vi "FRIC_navX_Internal_SPI_ProcessingLoop.vi"(7 "Device Number":T2, 11 "Rate (4Hz-200Hz)":u8=50 min=4 max=200) -> ()   [LabVIEW 2016, in "navX Library.lvlib"]
doc: "This navX VI handles the reading/writing for the navX. All of the good stuff is in here.\nTHIS VI SHOULD NOT BE CALLED BY THE USER!"
uses:
  navX Library.lvlib
  <vilib>/Rock Robotics/SystemInterfaces/spilib/spi_bus.ctl
  _TypeDefs/FRIC_navX_DeviceNumbersTypeDef.ctl
  _TypeDefs/FRIC_navX_I2C Process Loop TypeDef.ctl
  _TypeDefs/FRIC_navX_ProcessingLoopStatesTypeDef_I2C.ctl
  _TypeDefs/Z900_navX_DeviceTypeDef.ctl
  _TypeDefs/Z900_navX_ProtocolTypeDef.ctl
  _TypeDefs/Z900_navX_NotifyPacketTypeDef.ctl
  _TypeDefs/Z900_navX_ActionTypeDef.ctl
  _TypeDefs/Z900_navX_SerialStreamTypeDef.ctl
  <vilib>/Rock Robotics/SystemInterfaces/i2clib/i2c_bus.ctl
  _TypeDefs/Z900_navX_IntegrationControlRegisters.ctl
  <vilib>/Rock Robotics/WPI/SPI/WPI_SPIDevRef.ctl
  <vilib>/Rock Robotics/WPI/SerialPort/WPI_SerialPort.ctl
  <vilib>/Rock Robotics/WPI/SerialPort/WPI_SerialPortRef.ctl
  <vilib>/Platform/TimedLoop/XDataNode/timing_clust.ctl
  <vilib>/Platform/TimedLoop/XDataNode/nitl_modes.ctl
  <vilib>/Platform/TimedLoop/XDataNode/wakeup.ctl
  _TypeDefs/Flags/Z900_navX_Flags_CapabilityTypeDef.ctl
  _TypeDefs/Z900_navX_DeviceRegisters.ctl
  _Util/Z900_navX_Util_LittleEndian_to_BigEndian.vi
  <vilib>/Rock Robotics/SystemInterfaces/Utilities/FPGA_UtilitiesRead LocalTime.vi
  <vilib>/Platform/TimedLoop/XDataNode/XDataNode.xnode
  <vilib>/Platform/TimedLoop/XDataNode/XDNodeRunTimeDep.lvlib
panel:
  in  "Tab Control":enum32{"Page 1", "Page 2"}(tab)
  in  "Halt":bool
  out "Connected":bool
  in  "SPI Bus":T1=enum."SPI MXP"
  in  "Clock Rate (Hz)":dbl=2000000.0 format="%_6f"
  out "error":errorcluster
  out "Loop dt":i64
  out "Loop TIme":i64
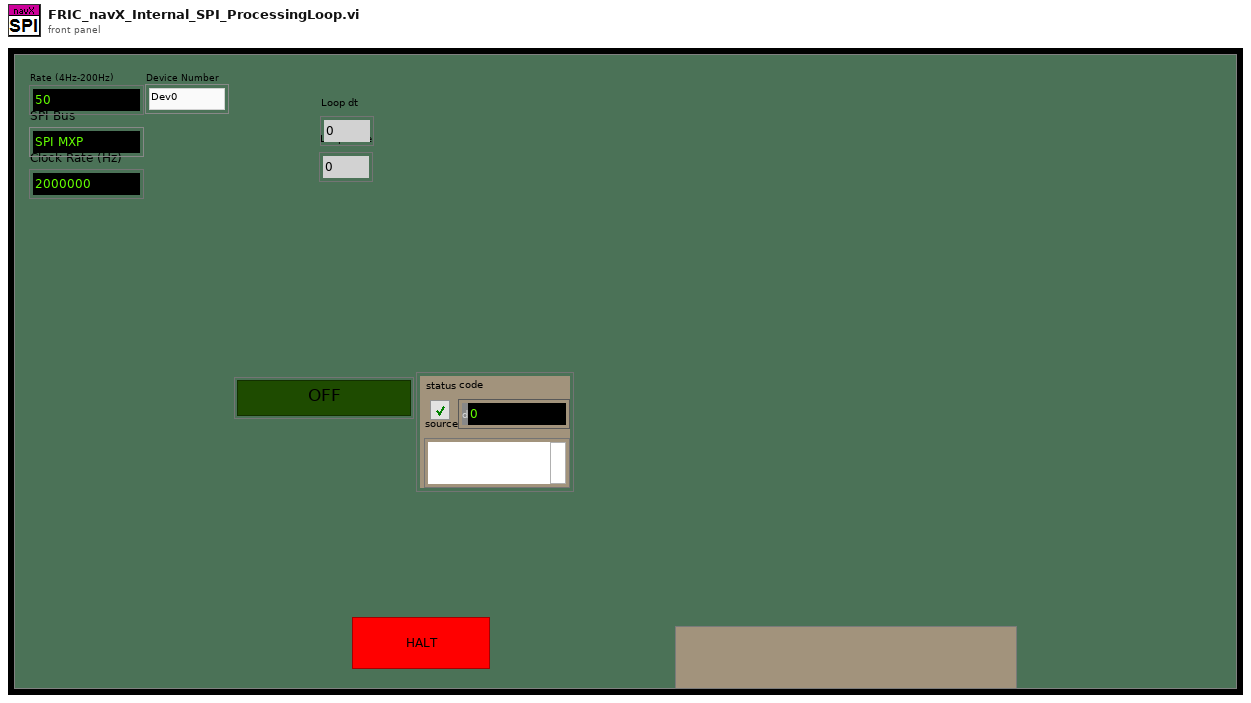
[diagram p1: front panel]
types:
  T1 = typedef "spi_bus.ctl" = enum16{"SPI On-Board, CS0", "SPI On-Board, CS1", "SPI On-Board, CS2", "SPI On-Board, CS3", "SPI MXP", "Invalid"}
  T2 = typedef "navX Library.lvlib/FRIC_navX_DeviceNumbersTypeDef.ctl" = enum16{"Dev0", "Dev1", "Dev2", "Dev3"}
  T3 = typedef "navX Library.lvlib/FRIC_navX_I2C Process Loop TypeDef.ctl" = cluster{"State Array":T4[], "error":errorcluster, "FPGA Cluster":cluster{"Last Valid FPGA Time":dbl, "Error Count":i32, "Initialized":bool}, "Device Info":T5, "I2CDevRef":cluster{"DevStatus":errorcluster, "Device Address":u8, "Handle":i32, "I2C Bus":T7}, "Registry":u8[], "Command Array":T8[], "Connected?":bool, "navX Device Memory Size":i32, "notification":T9, "Memory Size Set":bool, "SPIDevRef":T12, "navX Serial Open":cluster{"Stream Type":T11, "Serial Port":T13}, "SerialPortRef":T14, "Serial Read Buffer":string, "Serial Write Buffer":string[], "Device Number":T2, "navX SPI Open":cluster{"SPI Bus":T1, "Clock Rate (Hz)":dbl}, "Loop dt":i64, "current time":timestamp, "Loop Time":i64}
  T4 = typedef "navX Library.lvlib/FRIC_navX_ProcessingLoopStatesTypeDef_I2C.ctl" = enum16{"Process", "INI", "Check Packets Valid", "Close", "Clear VISA", "Generate Command", "Last Packet Valid", "Open", "Read", "Reset Serial", "Set Termination Char", "Update AE", "Wait", "Write", "Exit"}
  T5 = typedef "navX Library.lvlib/Z900_navX_DeviceTypeDef.ctl" = cluster{"Interface":cluster{"Protocol":T6, "Update Rate (4Hz-200Hz)":u8, "navX Open TypeDef":variant}, "Notify Packet":refnum<notifier>, "Loop VI Refnum":refnum<vi>, "Ready to Close Occurrence Refnum":refnum<k4>, "Name":string}
  T6 = typedef "navX Library.lvlib/Z900_navX_ProtocolTypeDef.ctl" = enum16{"SERIAL", "I2C", "SPI"}
  T7 = typedef "i2c_bus.ctl" = enum16{"I2C On-Board", "I2C MXP", "Invalid"}
  T8 = typedef "navX Library.lvlib/Z900_navX_IntegrationControlRegisters.ctl" = u8
  T9 = typedef "navX Library.lvlib/Z900_navX_NotifyPacketTypeDef.ctl" = cluster{"navX Action":T10, "Data":variant, "Stream Type":T11, "Device Number":T2}
  T10 = typedef "navX Library.lvlib/Z900_navX_ActionTypeDef.ctl" = enum16{"None", "Halt", "Normal Read", "Update Serial Protocol", "Update Rate Htz", "Zero-Yaw", "Zero-Displacement", "Zero-Velocity"}
  T11 = typedef "navX Library.lvlib/Z900_navX_SerialStreamTypeDef.ctl" = enum16{"YRPH", "Quaterinons", "Gyro/Raw", "AHRS", "AHRSAndPositioning", "AHRSAndPOSTime"}
  T12 = typedef "WPI_SPIDevRef.ctl" = cluster{"DevStatus":errorcluster, "Handle":i32, "SPI Bus":T1}
  T13 = typedef "WPI_SerialPort.ctl" = enum16{"Onboard RS-232", "MXP TTL", "USB 1", "USB 2"}
  T14 = typedef "WPI_SerialPortRef.ctl" = cluster{"DevStatus":errorcluster, "Serial Port Name":refnum<visa-resource-name>}
  T15 = typedef "XDNodeRunTimeDep.lvlib/timing_clust.ctl" = cluster{"Expected End [f-1]":u64, "Actual End [f-1]":u64, "Finished Late? [f-1]":bool, "Expected End [i-1]":u64, "Actual End [i-1]":u64, "Finished Late? [i-1]":bool, "Expected Start [i]":u64, "Actual Start [i]":u64, "Expected Start [f]":u64, "Actual Start [f]":u64, "Source Name":string, "Structure Name":string, "Period":i64, "Deadline":i64, "Offset":i64, "Start":i64, "Priority":i32, "Timeout":i32, "Mode":T16, "Wakeup Reason":T17, "Error":errorcluster, "Source Type":string, "Secondary Source Type":string, "Global End Time":u64, "Global Start Time":u64, "Frame Duration":u64, "Iteration Duration":u64, "Assigned CPU":i32, "I/O Scan Engine Mode":u32}
  T16 = typedef "XDNodeRunTimeDep.lvlib/nitl_modes.ctl" = enum32{"No Change", "Process missed periods, maintain original phase", "Discard missed periods, maintain original phase", "Process missed periods, ignore original phase", "Discard missed periods, ignore original phase"}
  T17 = typedef "XDNodeRunTimeDep.lvlib/wakeup.ctl" = enum32{"Normal", "Aborted", "Asynchronous wakeup", "Timing source error", "Timed loop error", "Timeout"}
  T18 = typedef "navX Library.lvlib/Z900_navX_DeviceRegisters.ctl" = u8
  T19 = typedef "navX Library.lvlib/Z900_navX_Flags_CapabilityTypeDef.ctl" = u16
  T20 = cluster{"Last Valid FPGA Time":dbl, "Error Count":i32, "Initialized":bool}
  T21 = typedef "Z900_navX_NotifyPacketTypeDef.ctl" = cluster{"navX Action":T22, "Data":variant, "Stream Type":T23, "Device Number":T24}
  T22 = typedef "Z900_navX_ActionTypeDef.ctl" = enum16{"None", "Halt", "Normal Read", "Update Serial Protocol", "Update Rate Htz", "Zero-Yaw", "Zero-Displacement", "Zero-Velocity"}
  T23 = typedef "Z900_navX_SerialStreamTypeDef.ctl" = enum16{"YRPH", "Quaterinons", "Gyro/Raw", "AHRS", "AHRSAndPositioning", "AHRSAndPOSTime"}
  T24 = typedef "FRIC_navX_DeviceNumbersTypeDef.ctl" = enum16{"Dev0", "Dev1", "Dev2", "Dev3"}
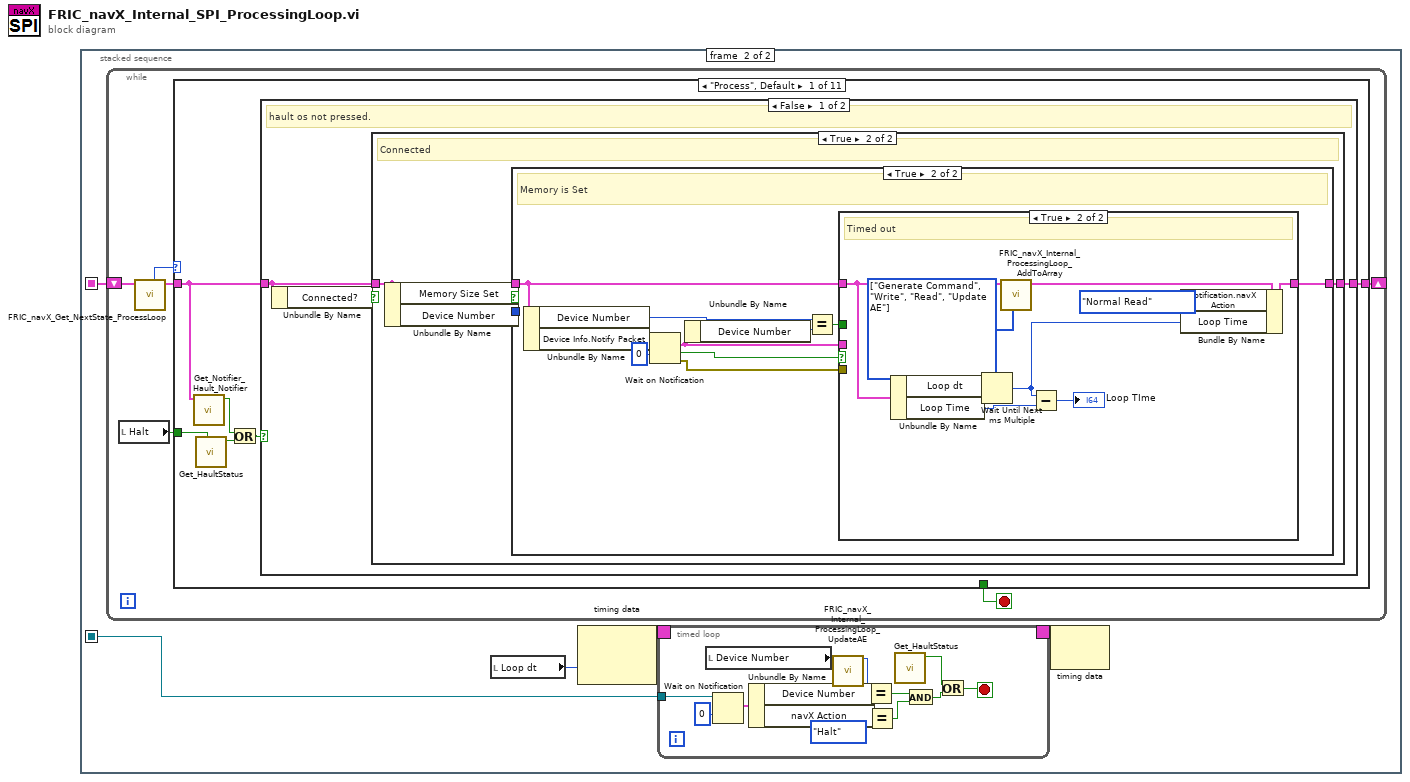
[diagram p0: block diagram]
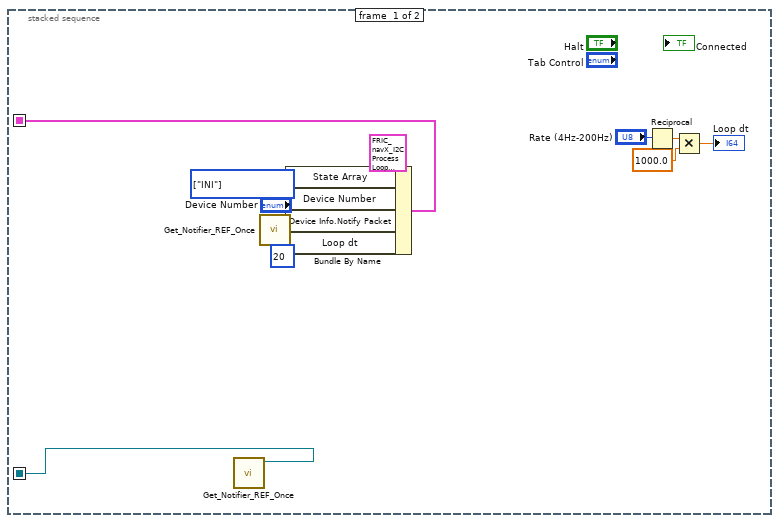
[diagram p2: hidden frame]
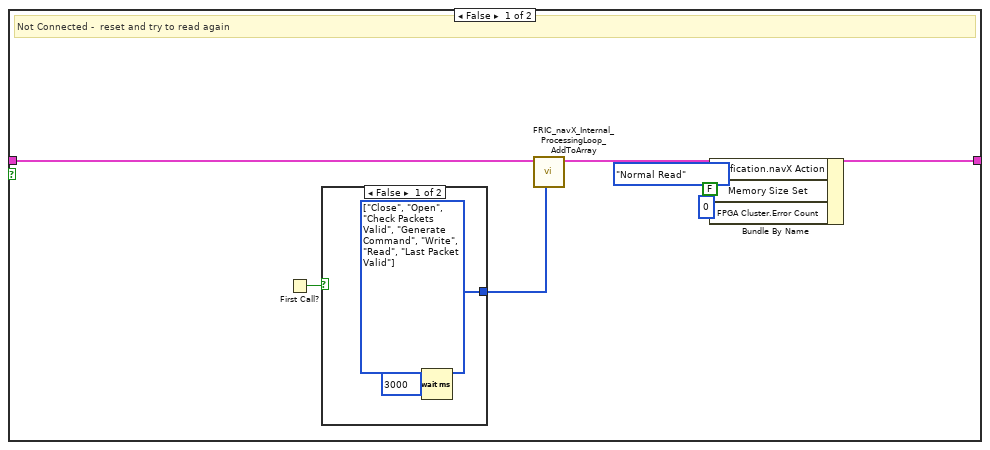
[diagram p3: hidden frame]
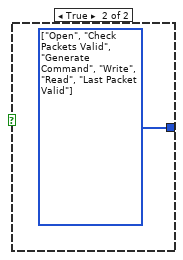
[diagram p4: hidden frame]
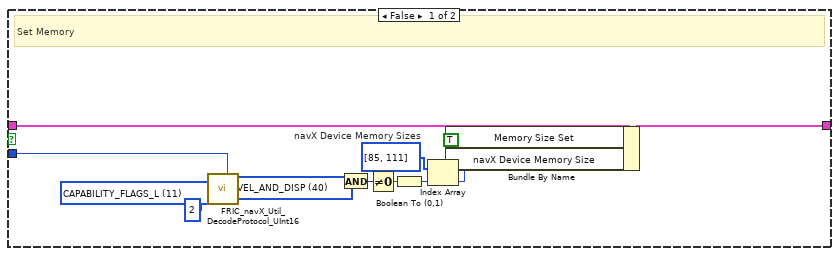
[diagram p5: hidden frame]
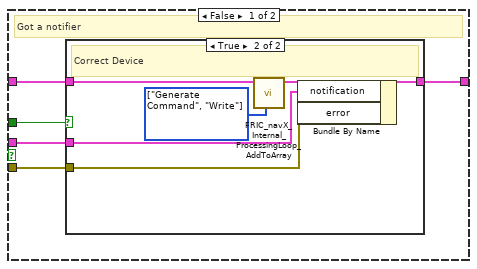
[diagram p6: hidden frame]
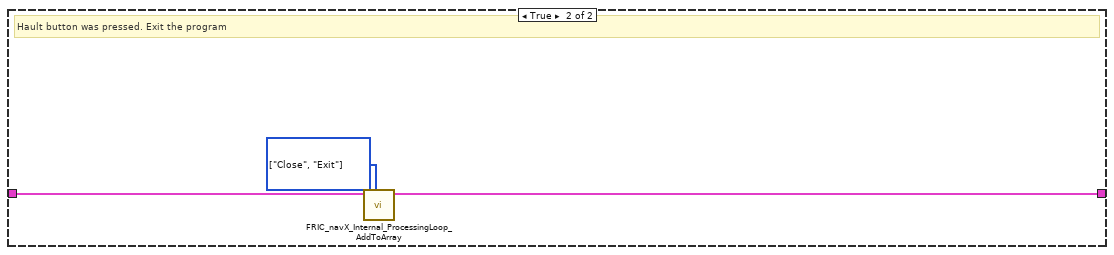
[diagram p8: hidden frame]
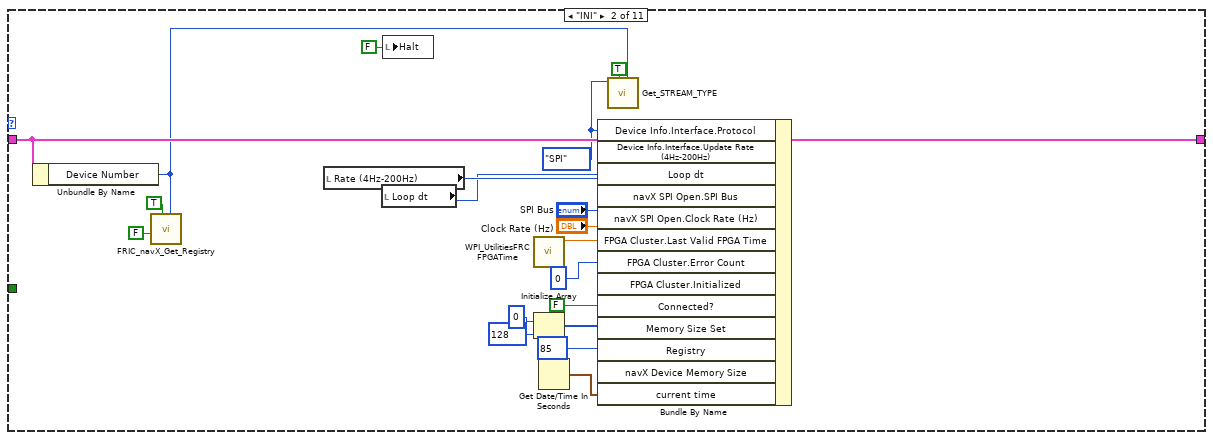
[diagram p9: hidden frame]
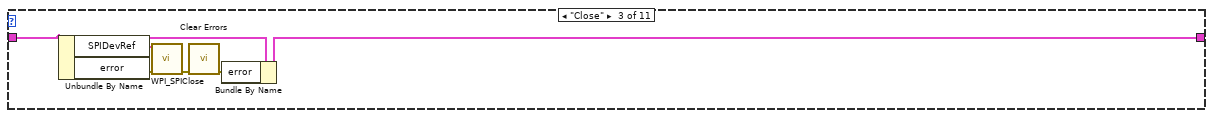
[diagram p10: hidden frame]
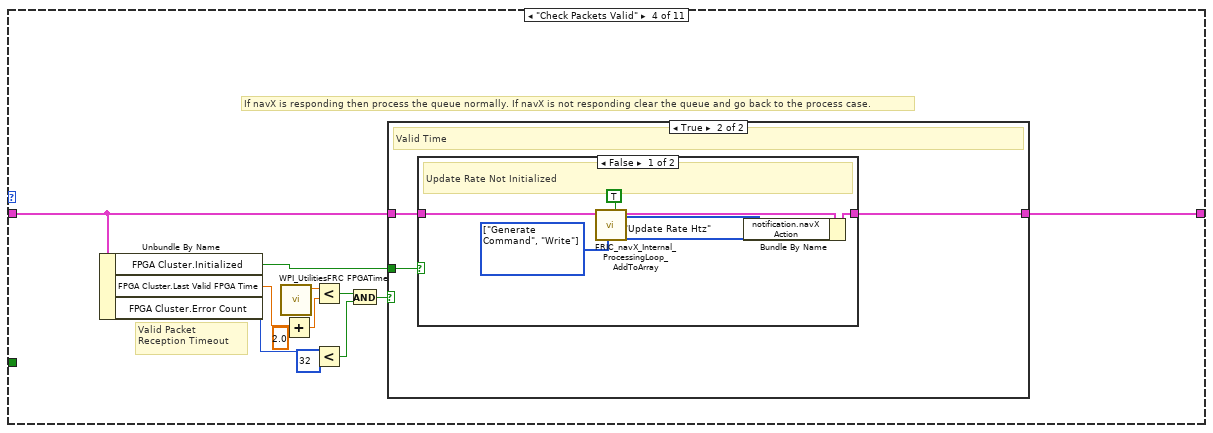
[diagram p11: hidden frame]
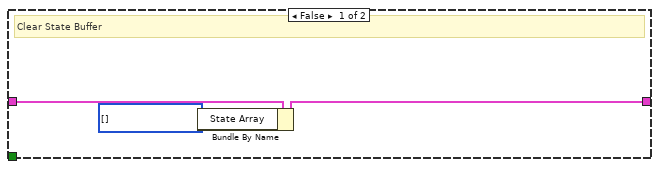
[diagram p12: hidden frame]
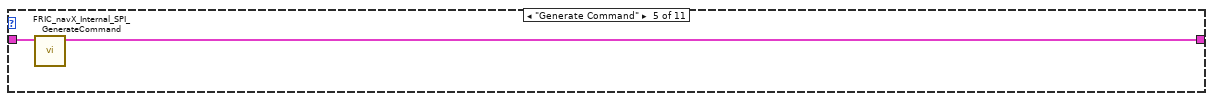
[diagram p14: hidden frame]
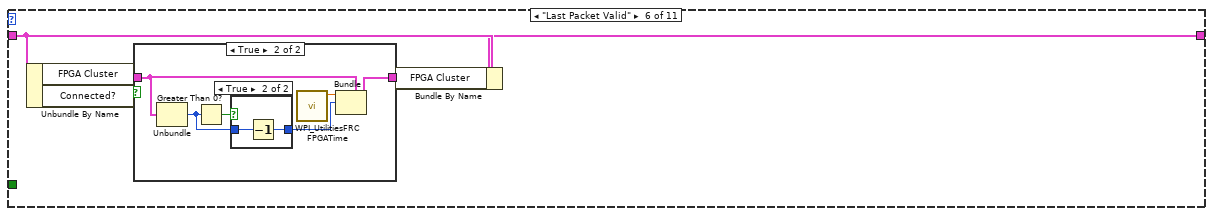
[diagram p15: hidden frame]
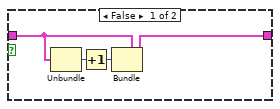
[diagram p16: hidden frame]
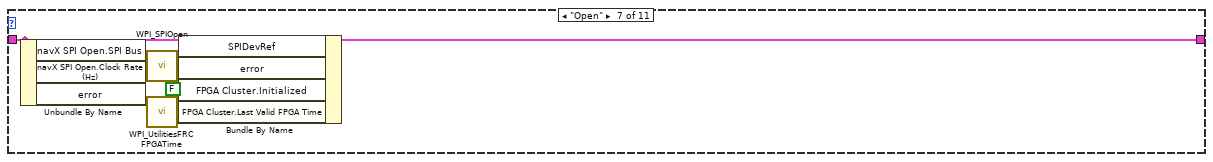
[diagram p18: hidden frame]
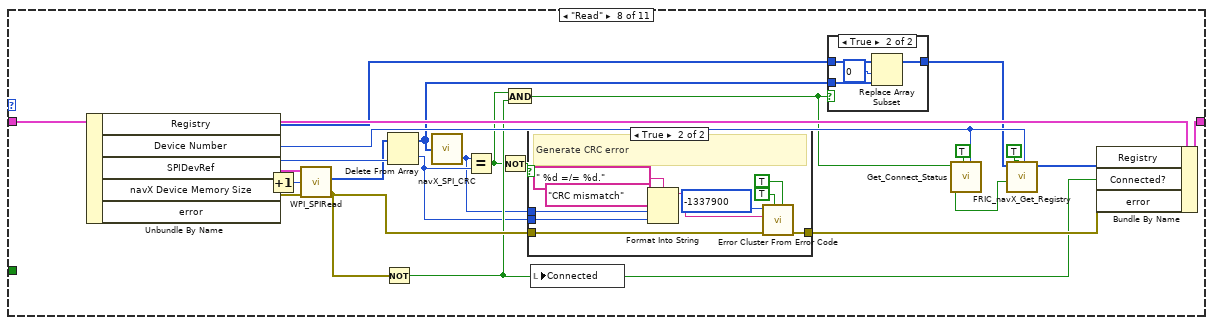
[diagram p19: hidden frame]
diagram:
  n1 = stacked-sequence {
    seq-local: [w11 _] -> [_ w16]
    seq-local: [w5 _] -> [_ w15]
    frame #0 {
      w9 = T4[] [enum."INI"] items=["Process", "INI", "Check Packets Valid", "Close", "Clear VISA", "Generate Command", "Last Packet Valid", "Open", "Read", "Reset Serial", "Set Termination Char", "Update AE", "Wait", "Write", "Exit"] ("State Array")
      n2 = call "Get_Notifier_REF_Once.vi"() -> ("notifier ref out"=w5:refnum<notifier>)  [unwired: 10 in, 1 out]
      n3 = call "Get_Notifier_REF_Once.vi"() -> ("notifier ref out"=w7:refnum<notifier>)  [unwired: 10 in, 1 out]
      n4 = Bundle By Name(cluster=T3 {"State Array"=[enum."INI", enum."Open"], "error"={"status"=FALSE, "code"=0, "source"=""}, "FPGA Cluster"={"Last Valid FPGA Time"=0.0, "Error Count"=0, "Initialized"=FALSE}, "Device Info"={"Interface"={"Protocol"=enum."SERIAL", "Update Rate (4Hz-200Hz)"=4, "navX Open TypeDef"=variant}, "Notify Packet"=refnum, "Loop VI Refnum"=refnum, "Ready to Close Occurrence Refnum"=refnum, "Name"=""}, "I2CDevRef"={"DevStatus"={"status"=FALSE, "code"=0, "source"=""}, "Device Address"=0, "Handle"=0, "I2C Bus"=enum."Invalid"}, "Registry"=[], "Command Array"=[214, 32], "Connected?"=FALSE, "navX Device Memory Size"=85, "notification"={"navX Action"=enum."None", "Data"=variant, "Stream Type"=enum."YRPH", "Device Number"=enum."Dev0"}, "Memory Size Set"=FALSE, "SPIDevRef"={"DevStatus"={"status"=FALSE, "code"=0, "source"=""}, "Handle"=0, "SPI Bus"=enum."SPI On-Board, CS0"}, "navX Serial Open"={"Stream Type"=enum."YRPH", "Serial Port"=enum."Onboard RS-232"}, "SerialPortRef"={"DevStatus"={"status"=FALSE, "code"=0, "source"=""}, "Serial Port Name"=""}, "Serial Read Buffer"="", "Serial Write Buffer"=[], "Device Number"=enum."Dev0", "navX SPI Open"={"SPI Bus"=enum."SPI MXP", "Clock Rate (Hz)"=500000.0}, "Loop dt"=0, "current time"=timestamp(0 s since 1904-01-01), "Loop Time"=0} ("I2C Process Loop TypeDef"), "State Array"=w9, "Device Number"="Device Number", "Device Info.Notify Packet"=w7, "Loop dt"=i64 20) -> (w11:T3)
      n5 = Reciprocal(x="Rate (4Hz-200Hz)") -> (1/x=w2:dbl)
      n6 = Multiply(x=w2, y=1000.0) -> (x*y=→"Loop dt":dbl)
    }
    frame #1 {
      n7 = while {
        shift-right: [w36] -> _
        shift-left: w16 -> [w39]
        stop <- w40 stop-if-true
        n8 = local read "Halt"() -> (w35:bool)
        n9 = call "FRIC_navX_Get_NextState_ProcessLoop.vi"("I2C Process Loop TypeDef (in)"=w39) -> ("I2C Process Loop TypeDef (out)"=w38:T3, "Current State"=w37:T4)  [unwired: 9 in]
        n10 = case shown="\"Process\", Default" w37 {
          tunnel: [_ _ _ _ _ _ _ _ _ w240 _] -> w40
          tunnel: w38 -> [w45 w120 w137 w141 w164 w168 w191 w213 w237 w242 w250]
          tunnel: [w46 w126 w136 w142 w163 w167 w190 w212 w230 w242 w250] -> w36
          tunnel: w35 -> [w43 _ _ _ _ _ _ _ _ _ _]
          frame "Process", Default {
            n11 = call "Get_Notifier_Hault_Notifier.vi"("Process Loop TypeDef (in)"=w45) -> ("Hault Notifier"=w41:bool)  [unwired: 10 in]
            n12 = call "Get_HaultStatus.vi"("Update"=w43) -> ("Hault"=w42:bool)  [unwired: 10 in]
            n13 = Or(x=w41, y=w42) -> (x .or. y?=w44:bool)
            n14 = case shown="False" w44 {
              tunnel: [w49 w110] -> w46
              tunnel: w45 -> [w47 w111]
              frame False {
                # "hault os not pressed."
                n15 = Unbundle By Name(w47) -> ("Connected?"=w48:bool)
                n16 = case shown="True" w48 {
                  tunnel: w47 -> [w57 w63]
                  tunnel: [w54 w64] -> w49
                  frame False {
                    # "Not Connected -  reset and try to read again"
                    n17 = First Call?() -> (First Call?: T/F=w50:bool)
                    n18 = case shown="False" w50 {
                      tunnel: [w59 w60] -> w56
                      frame False {
                        w59 = T4[] [enum."Close", enum."Open", enum."Check Packets Valid", enum."Generate Command", enum."Write", enum."Read", enum."Last Packet Valid"] items=["Process", "INI", "Check Packets Valid", "Close", "Clear VISA", "Generate Command", "Last Packet Valid", "Open", "Read", "Reset Serial", "Set Termination Char", "Update AE", "Wait", "Write", "Exit"]
                        n19 = Wait (ms)(milliseconds to wait=u32 3000) -> ()  [unwired: 1 out]
                      }
                      frame True {
                        w60 = T4[] [enum."Open", enum."Check Packets Valid", enum."Generate Command", enum."Write", enum."Read", enum."Last Packet Valid"] items=["Process", "INI", "Check Packets Valid", "Close", "Clear VISA", "Generate Command", "Last Packet Valid", "Open", "Read", "Reset Serial", "Set Termination Char", "Update AE", "Wait", "Write", "Exit"]
                      }
                    }
                    n20 = call "FRIC_navX_Internal_ProcessingLoop_AddToArray.vi"("States Array"=w56, "I2C Process Loop TypeDef (in)"=w57) -> ("I2C Process Loop TypeDef (out)"=w55:T3)  [unwired: 9 in]
                    n21 = Bundle By Name(cluster=w55, "notification.navX Action"=Z900_navX_ActionTypeDef."Normal Read", "Memory Size Set"=FALSE, "FPGA Cluster.Error Count"=0) -> (w54:T3)
                  }
                  frame True {
                    # "Connected"
                    n22 = Unbundle By Name(w63) -> ("Memory Size Set"=w62:bool, "Device Number"=w61:T2)
                    n23 = case shown="True" w62 {
                      tunnel: [w76 w85] -> w64
                      tunnel: w63 -> [w77 w83]
                      tunnel: w61 -> [w65 _]
                      frame False {
                        w75 = T18 11 items=["WHOAMI"=0, "HW_REV"=1, "FW_VER_MAJOR"=2, "FW_VER_MINOR"=3, "UPDATE_RATE_HZ"=4, "ACCEL_FSR_G"=5, "GYRO_FSR_DPS"=6, "OP_STATUS"=8, "CAL_STATUS"=9, "SELFTEST_STATUS"=10, "CAPABILITY_FLAGS_L"=11, "CAPABILITY_FLAGS_H"=12, "SENSOR_STATUS"=16, "TIMESTAMP"=18, "YAW"=22, "ROLL"=24, "PITCH"=26, "HEADING"=28, "FUSED_HEADING"=30, "ALTITUDE_I"=32, "ALTITUDE_D"=34, "LINERA_ACC_X"=36, "LINERA_ACC_Y"=38, "LINERA_ACC_Z"=40, "QUAT_W"=42, "QUAT_X"=44, "QUAT_Y"=46, "QUAT_Z"=48, "MPU_TEMP_C"=50, "GYRO_X"=52, "GYRO_Y"=54, "GYRO_Z"=56, "ACC_X"=58, "ACC_Y"=60, "ACC_Z"=62, "MAG_X"=64, "MAG_Y"=66, "MAG_Z"=68, "PRESSURE_I"=70, "PRESSURE_D"=72, "PRESSURE_TEMP"=74, "YAW_OFFSET"=76, "QUAT_OFFSET_W"=78, "QUAT_OFFSET_X"=80, "QUAT_OFFSET_Y"=82, "QUAT_OFFSET_Z"=84, "INTEGRATION_CONTROL"=86, "VELOCITY_X"=88, "VELOCITY_Y"=92, "VELOCITY_Z"=96, "DISPLACMENT_X"=100, "DISPLACMENT_Y"=104, "DISPLACEMENT_Z"=108] ("Device Register")
                        w70 = T19 40 items=["OMNIMOUNT"=4, "OMNIMOUNT_CONFIG_MASK"=38, "VEL_AND_DISP"=40, "YAW_RESET"=80] ("Capability Flag")
                        w71 = i32[] [85, 111]  # navX Device Memory Sizes
                        # "Set Memory"
                        n24 = call "FRIC_navX_Util_DecodeProtocol_UInt16.vi"("Device Number"=w65, "length"=2, "Device Register"=w75) -> ("Value"=w68:u16)  [unwired: 8 in]
                        n25 = And(x=w68, y=w70) -> (x .and. y?=w69:T19)
                        n26 = Not Equal To 0?(x=w69) -> (x != 0?=w72:bool)
                        n27 = Boolean To (0,1)(Boolean=w72) -> (0, 1=w73:i16)
                        n28 = Index Array(array=w71, index=w73) -> (element=w66:i32)
                        n29 = Bundle By Name(cluster=w77, "Memory Size Set"=TRUE, "navX Device Memory Size"=w66) -> (w76:T3)
                      }
                      frame True {
                        # "Memory is Set"
                        n30 = Unbundle By Name(w83) -> ("Device Number"=w80:T2, "Device Info.Notify Packet"=w87:refnum<notifier>)
                        n31 = Wait on Notification(notifier=w87, timeout in ms (-1)=0) -> (notification=w81:T9, timed out?=w82:bool, error out=w84:errorcluster)  [unwired: 2 in, 1 out]
                        n32 = Unbundle By Name(w81) -> ("Device Number"=w79:T2)
                        n33 = Equal?(x=w80, y=w79) -> (x = y?=w78:bool)
                        n34 = case shown="True" w82 {
                          tunnel: w83 -> [w92 w104]
                          tunnel: [w91 w106] -> w85
                          tunnel: w81 -> [w90 _]
                          tunnel: w84 -> [w89 _]
                          tunnel: w78 -> [w88 _]
                          frame False {
                            # "Got a notifier"
                            n35 = case shown="True" w88 {
                              tunnel: w92 -> [w93 w99]
                              tunnel: [w93 w98] -> w91
                              tunnel: w90 -> [_ w97]
                              tunnel: w89 -> [_ w94]
                              frame False {
                              }
                              frame True {
                                w95 = T4[] [enum."Generate Command", enum."Write"] items=["Process", "INI", "Check Packets Valid", "Close", "Clear VISA", "Generate Command", "Last Packet Valid", "Open", "Read", "Reset Serial", "Set Termination Char", "Update AE", "Wait", "Write", "Exit"] ("States Array")
                                # "Correct Device"
                                n36 = call "FRIC_navX_Internal_ProcessingLoop_AddToArray.vi"("States Array"=w95, "I2C Process Loop TypeDef (in)"=w99) -> ("I2C Process Loop TypeDef (out)"=w96:T3)  [unwired: 9 in]
                                n37 = Bundle By Name(cluster=w96, "notification"=w97, "error"=w94) -> (w98:T3)
                              }
                            }
                          }
                          frame True {
                            w108 = T4[] [enum."Generate Command", enum."Write", enum."Read", enum."Update AE"] items=["Process", "INI", "Check Packets Valid", "Close", "Clear VISA", "Generate Command", "Last Packet Valid", "Open", "Read", "Reset Serial", "Set Termination Char", "Update AE", "Wait", "Write", "Exit"]
                            # "Timed out"
                            n38 = Unbundle By Name(w104) -> ("Loop dt"=w101:i64, "Loop Time"=w100:i64)
                            n39 = Wait Until Next ms Multiple(millisecond multiple=w101) -> (millisecond timer value=w102:u32)
                            n40 = call "FRIC_navX_Internal_ProcessingLoop_AddToArray.vi"("States Array"=w108, "I2C Process Loop TypeDef (in)"=w104) -> ("I2C Process Loop TypeDef (out)"=w107:T3)  [unwired: 9 in]
                            n41 = Subtract(x=w102, y=w100) -> (x-y=→"Loop TIme":i64)
                            n42 = Bundle By Name(cluster=w107, "notification.navX Action"=Z900_navX_ActionTypeDef."Normal Read", "Loop Time"=w102) -> (w106:T3)
                          }
                        }
                      }
                    }
                  }
                }
              }
              frame True {
                w109 = T4[] [enum."Close", enum."Exit"] items=["Process", "INI", "Check Packets Valid", "Close", "Clear VISA", "Generate Command", "Last Packet Valid", "Open", "Read", "Reset Serial", "Set Termination Char", "Update AE", "Wait", "Write", "Exit"] ("States Array")
                # "Hault button was pressed. Exit the program"
                n43 = call "FRIC_navX_Internal_ProcessingLoop_AddToArray.vi"("States Array"=w109, "I2C Process Loop TypeDef (in)"=w111) -> ("I2C Process Loop TypeDef (out)"=w110:T3)  [unwired: 9 in]
              }
            }
          }
          frame "INI" {
            w112 = Z900_navX_ProtocolTypeDef."SPI" ("Protocol")
            w124 = FALSE ("Initialized")
            n44 = Unbundle By Name(w120) -> ("Device Number"=w113:T2)
            n45 = call "FRIC_navX_Get_Registry.vi"("Device Number"=w113, "Update"=TRUE, "Connected?"=FALSE) -> ()  [unwired: 7 in, 2 out]
            n46 = local read "Rate (4Hz-200Hz)"() -> (w116:u8)
            n47 = local read "Loop dt"() -> (w115:i64)
            n48 = local write "Halt"(FALSE ("Halt")) -> ()
            n49 = call <vilib>:"WPI_UtilitiesFRC FPGATime.vi"() -> ("FPGA Time"=w128:dbl)  [unwired: 10 in, 1 out]
            n50 = Initialize Array(u8 0 ("Received Data"), 128 ("hex")) -> (w122:u8[])
            n51 = Get Date/Time In Seconds() -> (seconds since 1Jan1904=w117:timestamp)
            n52 = Bundle By Name(cluster=w120, "Device Info.Interface.Protocol"=w112, "Device Info.Interface.Update Rate (4Hz-200Hz)"=w116, "Loop dt"=w115, "navX SPI Open.SPI Bus"="SPI Bus", "navX SPI Open.Clock Rate (Hz)"="Clock Rate (Hz)", "FPGA Cluster.Last Valid FPGA Time"=w128, "FPGA Cluster.Error Count"=0 ("Error Count"), "FPGA Cluster.Initialized"=w124, "Connected?"=w124, "Memory Size Set"=w124, "Registry"=w122, "navX Device Memory Size"=85 ("hex"), "current time"=w117) -> (w126:T3)
            n53 = call "Get_STREAM_TYPE.vi"("Device Number"=w113, "Update"=TRUE, "Protocol (in)"=w112) -> ()  [unwired: 8 in, 1 out]
          }
          frame "Close" {
            n54 = Unbundle By Name(w137) -> ("SPIDevRef"=w135:T12, "error"=w134:errorcluster)
            n55 = call <vilib>:"WPI_SPIClose.vi"("error in (no error)"=w134, "SPIDevRef"=w135) -> ("error out"=w133:errorcluster)  [unwired: 9 in]
            n56 = call <vilib>:"Clear Errors.vi"("error in (no error)"=w133) -> ("error out"=w132:errorcluster)  [unwired: 5 in, 1 out]
            n57 = Bundle By Name(cluster=w137, "error"=w132) -> (w136:T3)
          }
          frame "Check Packets Valid" {
            # "If navX is responding then process the queue normally. If navX is not responding clear the queue and go back to the process case."
            # "Valid Packet Reception Timeout"
            n58 = Unbundle By Name(w141) -> ("FPGA Cluster.Initialized"=w139:bool, "FPGA Cluster.Last Valid FPGA Time"=w140:dbl, "FPGA Cluster.Error Count"=w138:i32)
            n59 = call <vilib>:"WPI_UtilitiesFRC FPGATime.vi"() -> ("FPGA Time"=w147:dbl)  [unwired: 10 in, 1 out]
            n60 = Add(x=w140, y=2.0) -> (x+y=w148:dbl)
            n61 = Less?(x=w147, y=w148) -> (x < y?=w145:bool)
            n62 = Less?(x=w138, y=32) -> (x < y?=w144:bool)
            n63 = And(x=w145, y=w144) -> (x .and. y?=w143:bool)
            n64 = case shown="True" w143 {
              tunnel: w141 -> [w152 w155]
              tunnel: [w151 w154] -> w142
              tunnel: w139 -> [_ w153]
              frame False {
                w150 = T4[] [] items=["Process", "INI", "Check Packets Valid", "Close", "Clear VISA", "Generate Command", "Last Packet Valid", "Open", "Read", "Reset Serial", "Set Termination Char", "Update AE", "Wait", "Write", "Exit"] ("f")
                # "Clear State Buffer"
                n65 = Bundle By Name(cluster=w152, "State Array"=w150) -> (w151:T3)
              }
              frame True {
                # "Valid Time"
                n66 = case shown="False" w153 {
                  tunnel: w155 -> [w160 w162]
                  tunnel: [w158 w162] -> w154
                  frame False {
                    w156 = T4[] [enum."Generate Command", enum."Write"] items=["Process", "INI", "Check Packets Valid", "Close", "Clear VISA", "Generate Command", "Last Packet Valid", "Open", "Read", "Reset Serial", "Set Termination Char", "Update AE", "Wait", "Write", "Exit"] ("f")
                    # "Update Rate Not Initialized"
                    n67 = call "FRIC_navX_Internal_ProcessingLoop_AddToArray.vi"("Add to beginning"=TRUE, "States Array"=w156, "I2C Process Loop TypeDef (in)"=w160) -> ("I2C Process Loop TypeDef (out)"=w159:T3)  [unwired: 8 in]
                    n68 = Bundle By Name(cluster=w159, "notification.navX Action"=Z900_navX_ActionTypeDef."Update Rate Htz") -> (w158:T3)
                  }
                  frame True {
                    # "Update Rate is Initialized"
                  }
                }
              }
            }
          }
          frame "Generate Command" {
            n69 = call "FRIC_navX_Internal_SPI_GenerateCommand.vi"("I2C Process Loop TypeDef (in)"=w164) -> ("I2C Process Loop TypeDef (out)"=w163:T3)  [unwired: 10 in]
          }
          frame "Last Packet Valid" {
            n70 = Unbundle By Name(w168) -> ("FPGA Cluster"=w169:T20, "Connected?"=w165:bool)
            n71 = case shown="True" w165 {
              tunnel: [w172 w179] -> w166
              tunnel: w169 -> [w171 w175]
              frame False {
                n72 = Unbundle(w171) -> ("Error Count"=w170:i32)  [unwired: 2 out]
                n73 = Increment(x=w170) -> (x+1=w173:i32)
                n74 = Bundle(cluster=w171, "Error Count"=w173) -> (w172:T20)  [unwired: 2 in]
              }
              frame True {
                n75 = Unbundle(w175) -> ("Error Count"=w174:i32)  [unwired: 2 out]
                n76 = Greater Than 0?(x=w174) -> (x > 0?=w177:bool)
                n77 = case shown="True" w177 {
                  tunnel: [w180 w182] -> w176
                  tunnel: w174 -> [w180 w181]
                  frame False {
                  }
                  frame True {
                    n78 = Decrement(x=w181) -> (x-1=w182:i32)
                  }
                }
                n79 = call <vilib>:"WPI_UtilitiesFRC FPGATime.vi"() -> ("FPGA Time"=w178:dbl)  [unwired: 10 in, 1 out]
                n80 = Bundle(cluster=w175, "Last Valid FPGA Time"=w178, "Error Count"=w176) -> (w179:T20)  [unwired: 1 in]
              }
            }
            n81 = Bundle By Name(cluster=w168, "FPGA Cluster"=w166) -> (w167:T3)
          }
          frame "Open" {
            n82 = Unbundle By Name(w191) -> ("navX SPI Open.SPI Bus"=w184:T1, "navX SPI Open.Clock Rate (Hz)"=w183:dbl, "error"=w185:errorcluster)
            n83 = call <vilib>:"WPI_SPIOpen.vi"("error in"=w185, "Clock Rate (Hz)"=w183, "SPI Bus"=w184) -> ("error out"=w187:errorcluster, "SPIDevRef"=w188:T12)  [unwired: 7 in]
            n84 = call <vilib>:"WPI_UtilitiesFRC FPGATime.vi"() -> ("FPGA Time"=w186:dbl)  [unwired: 10 in, 1 out]
            n85 = Bundle By Name(cluster=w191, "SPIDevRef"=w188, "error"=w187, "FPGA Cluster.Initialized"=FALSE ("Initialized"), "FPGA Cluster.Last Valid FPGA Time"=w186) -> (w190:T3)
          }
          frame "Read" {
            n86 = Unbundle By Name(w213) -> ("Registry"=w210:u8[], "Device Number"=w204:T2, "SPIDevRef"=w209:T12, "navX Device Memory Size"=w206:i32, "error"=w208:errorcluster)
            n87 = Increment(x=w206) -> (x+1=w205:i32)
            n88 = call <vilib>:"WPI_SPIRead.vi"("error in (no error)"=w208, "Num to Read"=w205, "SPIDevRef"=w209) -> ("error out"=w202:errorcluster, "Received Data"=w198:u8[])  [unwired: 6 in, 1 out]
            n89 = Not(x=w202) -> (.not. x?=w201:bool)
            n90 = Delete From Array(array=w198, index=w206) -> (deleted portion=w196:u8, array with subset deleted=w194:u8[])  [unwired: 1 in]
            n91 = call "navX_SPI_CRC.vi"("Message"=w194) -> ("CRC"=w193:u8)  [unwired: 1 out]
            n92 = Equal?(x=w193, y=w196) -> (x = y?=w197:bool)
            n93 = Not(x=w197) -> (.not. x?=w195:bool)
            n94 = And(x=w197, y=w201) -> (x .and. y?=w199:bool)
            n95 = case shown="True" w195 {
              tunnel: w193 -> [_ w222]
              tunnel: w196 -> [_ w221]
              tunnel: w202 -> [w214 w218]
              tunnel: [w214 w217] -> w207
              frame False {
              }
              frame True {
                # "Generate CRC error"
                n96 = Format Into String(format string=" %d =/= %d.", initial string="CRC mismatch", w222, w221) -> (resulting string=w219:string)  [unwired: 1 in, 1 out]
                n97 = call <vilib>:"Error Cluster From Error Code.vi"("is warning? (False)"=TRUE, "show call chain? (False)"=TRUE, "error in (no error)"=w218, "error message (\"\")"=w219, "error code (0)"=-1337900 ("code")) -> ("error out"=w217:errorcluster)  [unwired: 4 in]
              }
            }
            n98 = local write "Connected"(w201) -> ()
            n99 = case shown="True" w199 {
              tunnel: w210 -> [_ w229]
              tunnel: [w225 w228] -> w192
              tunnel: w194 -> [w225 w227]
              frame False {
              }
              frame True {
                n100 = Replace Array Subset(array=w229, new element=w227, index=u8 0 ("hex")) -> (w228:u8[])
              }
            }
            n101 = call "Get_Connect_Status.vi"("Device Number"=w204, "Update"=TRUE, "Connected"=w199) -> ()  [unwired: 8 in, 1 out]
            n102 = call "FRIC_navX_Get_Registry.vi"("Device Number"=w204, "Update"=TRUE, "Connected?"=w199, "Registry (in)"=w192) -> ("Registry (out)"=w211:u8[])  [unwired: 6 in, 1 out]
            n103 = Bundle By Name(cluster=w213, "Registry"=w211, "Connected?"=w201, "error"=w207) -> (w212:T3)
          }
          frame "Write" {
            n104 = Unbundle By Name(w237) -> ("SPIDevRef"=w236:T12, "Command Array"=w235:T8[], "I2CDevRef.DevStatus"=w234:errorcluster)
            n105 = call <vilib>:"WPI_SPIWrite.vi"("error in (no error)"=w234, "Data To Send"=w235, "SPIDevRef"=w236) -> ("error out"=w233:errorcluster, "SPIDevRef"=w232:T12)  [unwired: 6 in, 1 out]
            n106 = Bundle By Name(cluster=w237, "SPIDevRef"=w232, "error"=w233) -> (w231:T3)
            n107 = flat-sequence {
              tunnel: w231 -> [w239]
              tunnel: [w239] -> w230
              frame #0 {
                n108 = Wait (ms)(milliseconds to wait=u32 1) -> ()  [unwired: 1 out]
              }
            }
          }
          frame "Exit" {
            n109 = Unbundle By Name(w242) -> ("Device Info"=w241:T5)
            n110 = in-place {
              in-place-border: [TRUE] -> w240
              in-place-border: w241 -> [w243]
              # "Set Occurence of Close"
              n111 = Unbundle By Name(w243) -> ("Ready to Close Occurrence Refnum"=w245:refnum<k4>)
              n112 = local write "Halt"(FALSE ("Halt")) -> ()
              n113 = Set Occurrence(w245) -> ()
            }
          }
          frame "Update AE" {
            n114 = Unbundle By Name(w250) -> ("Device Number"=w247:T2, "error"=w249:errorcluster)
            "error" <- w249
            n115 = call "Get_Error_Status.vi"("Device Number"=w247, "Update"=TRUE, "error in"=w249) -> ()  [unwired: 8 in, 1 out]
          }
        }
      }
      n116 = local read "Loop dt"() -> (w12:i64)
      n117 = node-c288(w12) -> (w14:T15)  [unwired: 1 in]
      n118 = timed-loop {
        timing: w14 -> [_]
        timing-out: [_] -> w13
        tunnel: w15 -> [w25]
        stop <- w17 stop-if-true
        n119 = local read "Device Number"() -> (w22:T2)
        n120 = Wait on Notification(notifier=w25, timeout in ms (-1)=0) -> (notification=w24:T21)  [unwired: 2 in, 3 out]
        n121 = Unbundle By Name(w24) -> ("Device Number"=w23:T24, "navX Action"=w27:T22)
        n122 = call "FRIC_navX_Internal_ProcessingLoop_UpdateAE.vi"("Device Number"=w22) -> ()  [unwired: 15 in]
        n123 = Equal?(x=w22, y=w23) -> (x = y?=w21:bool)
        n124 = Equal?(x=w27, y=Z900_navX_ActionTypeDef."Halt") -> (x = y?=w20:bool)
        n125 = call "Get_HaultStatus.vi"() -> ("Hault"=w19:bool)  [unwired: 11 in]
        n126 = And(x=w21, y=w20) -> (x .and. y?=w18:bool)
        n127 = Or(x=w19, y=w18) -> (x .or. y?=w17:bool)
      }
      n128 = node-c288(w13) -> ()  [unwired: 1 out]
    }
  }
